vi "Circular.vi"(5 "Direction":u16(ring) items=["Clockwise", "Counter-clockwise"], 7 "Speed":dbl, 8 "error in (no error)":errorcluster, 9 "XY End":dbl[](array[numeric]), 10 "XY Center":dbl[](array[numeric]), 11 "Gantry In":refnum<k24>) -> (0 "error out":errorcluster, 3 "Gantry Out":refnum<k24>)   [LabVIEW 2020, in "A3200.lvclass"]
uses:
  A3200.lvclass
  C:/Program Files (x86)/Aerotech/A3200/LabVIEW/2010/Bin/Aerotech.A3200.dll
  Program Files (x86)/Aerotech/A3200/LabVIEW/2010/Bin/Aerotech.A3200.dll
  Drivers/Aerotech A3200/Aerotech VIs.lvlib
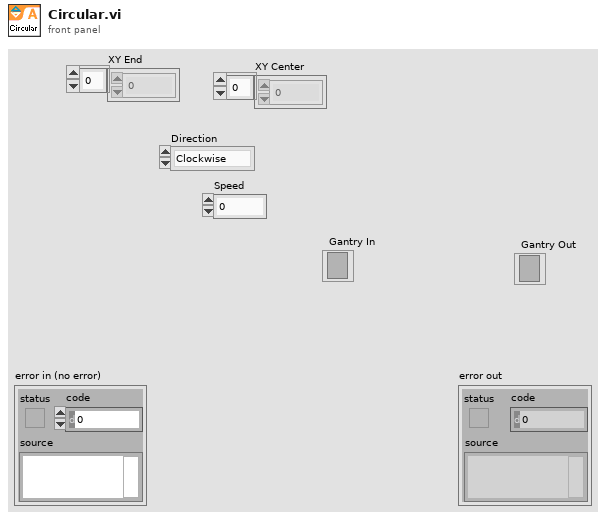
[diagram p1: front panel]
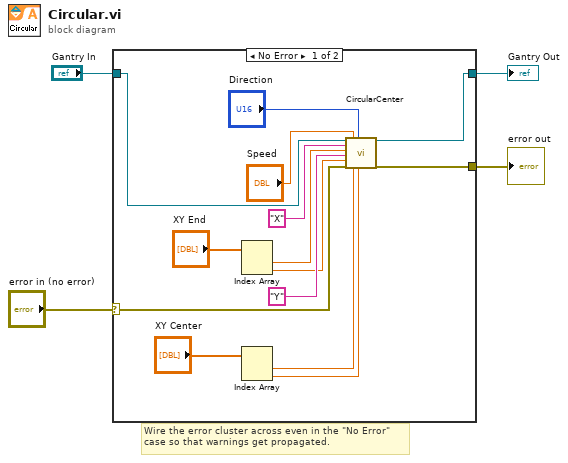
[diagram p0: block diagram]
diagram:
  # "Wire the error cluster across even in the \"No Error\"\ncase so that warnings get propagated."
  n1 = case shown="No Error" "error in (no error)" {
    selector: "error in (no error)" -> [w6 w20]
    tunnel: [w5 w20] -> w3
    tunnel: "Gantry In" -> [w8 w19]
    tunnel: [w7 w19] -> w1
    frame No Error {
      n2 = Index Array(array="XY End") -> (element #1=w12:dbl, element #2=w11:dbl)  [unwired: 2 in]
      n3 = Index Array(array="XY Center") -> (element #1=w16:dbl, element #2=w15:dbl)  [unwired: 2 in]
      n4 = call "CircularCenter.vi"("controller in"=w8, "axis 1 name"="X", "axis 1 endpoint"=w12, "axis 2 name"="Y" ("axis 1 name"), "axis 2 endpoint"=w11, "error in (no error)"=w6, "speed"="Speed", "axis 1 center point"=w16, "direction"="Direction", "axis 2 center point"=w15) -> ("controller out"=w7:refnum<k24>, "error out"=w5:errorcluster)  [unwired: 8 in]
    }
    frame Error {
    }
  }
  "error out" <- w3
  "Gantry Out" <- w1
